vi "总磷总氮流程质控自动启动.vi"(9 "总磷量程切换":enum32{"H", "L", "AUTO"}(ring)=enum."AUTO", 10 "总氮量程切换":enum32{"H", "L", "AUTO"}(ring)=enum."AUTO", 11 "参数":T1={"是否启用仪器"=FALSE, "CODMn"={"启动测量模式"={"测量模式"=enum."水样测量"}, "确定按钮"=TRUE}, "启动模块"={"氨氮"=FALSE, "总磷"=FALSE, "总氮"=FALSE, "COD"=FALSE}, "常规启动"=FALSE, "直接启动"=FALSE}) -> ()   [LabVIEW 2016, in "质控单元.lvlib"]
uses:
  PLC/PLC.lvlib
panel:
  out "枚举 2":enum16{"初始化", "采配水启动", "等待", "配水", "排水", "结束"}(ring)
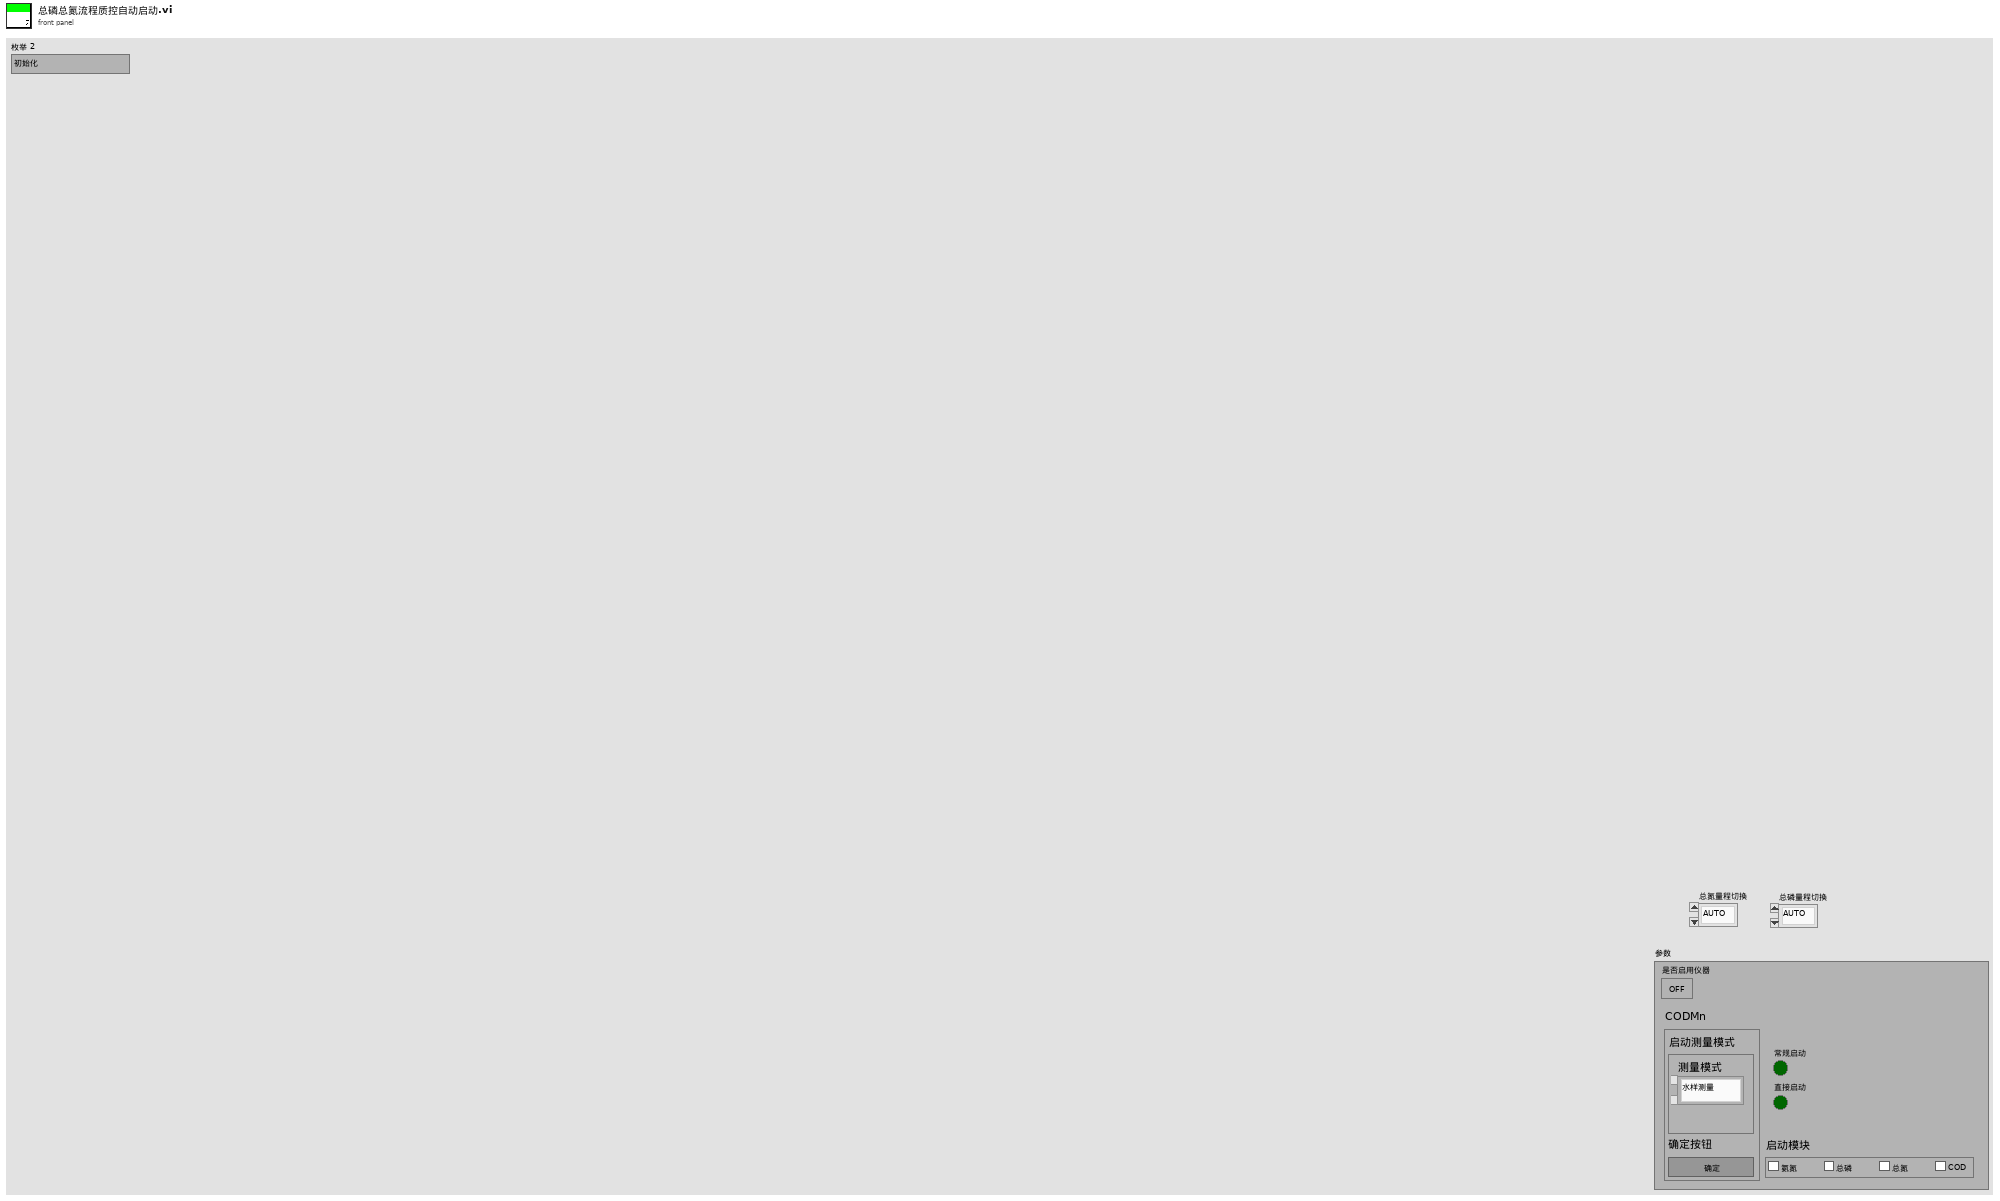
[diagram p1: front panel]
types:
  T1 = cluster{"是否启用仪器":bool, "CODMn":cluster{"启动测量模式":cluster{"测量模式":enum16{"水样测量", "标样核查", "加标回收", "平行样", "校零", "校标"}}, "确定按钮":bool}, "启动模块":cluster{"氨氮":bool, "总磷":bool, "总氮":bool, "COD":bool}, "常规启动":bool, "直接启动":bool}
  T2 = cluster{"R0":i16, "R1":i16, "R2":i16, "R3":i16, "R4":i16, "R5":i16, "R6":i16, "R7":i16, "R8":i16, "R9":i16, "R10":i16, "R11":i16, "R12":i16, "R13":i16, "R14":i16, "R15":i16, "R16":i16, "R17":i16, "R18":i16, "R19":i16, "R20":i16, "R21":i16, "R22":i16, "R23":i16, "R24":i16, "R25":i16, "R26":i16, "R27":i16, "R28":i16, "R29":i16, "R30":i16, "R31":i16, "R32":i16, "R33":i16, "R34":i16, "R35":i16, "R36":i16, "R37":i16, "R38":i16, "R39":i16, "R40":i16, "R41":i16, "R42":i16, "R43":i16, "R44":i16, "R45":i16, "R46":i16, "R47":i16, "R48":i16, "R49":i16, "R50":i16, "R51":i16, "R52":i16, "R53":i16, "R54":i16, "R55":i16, "R56":i16}
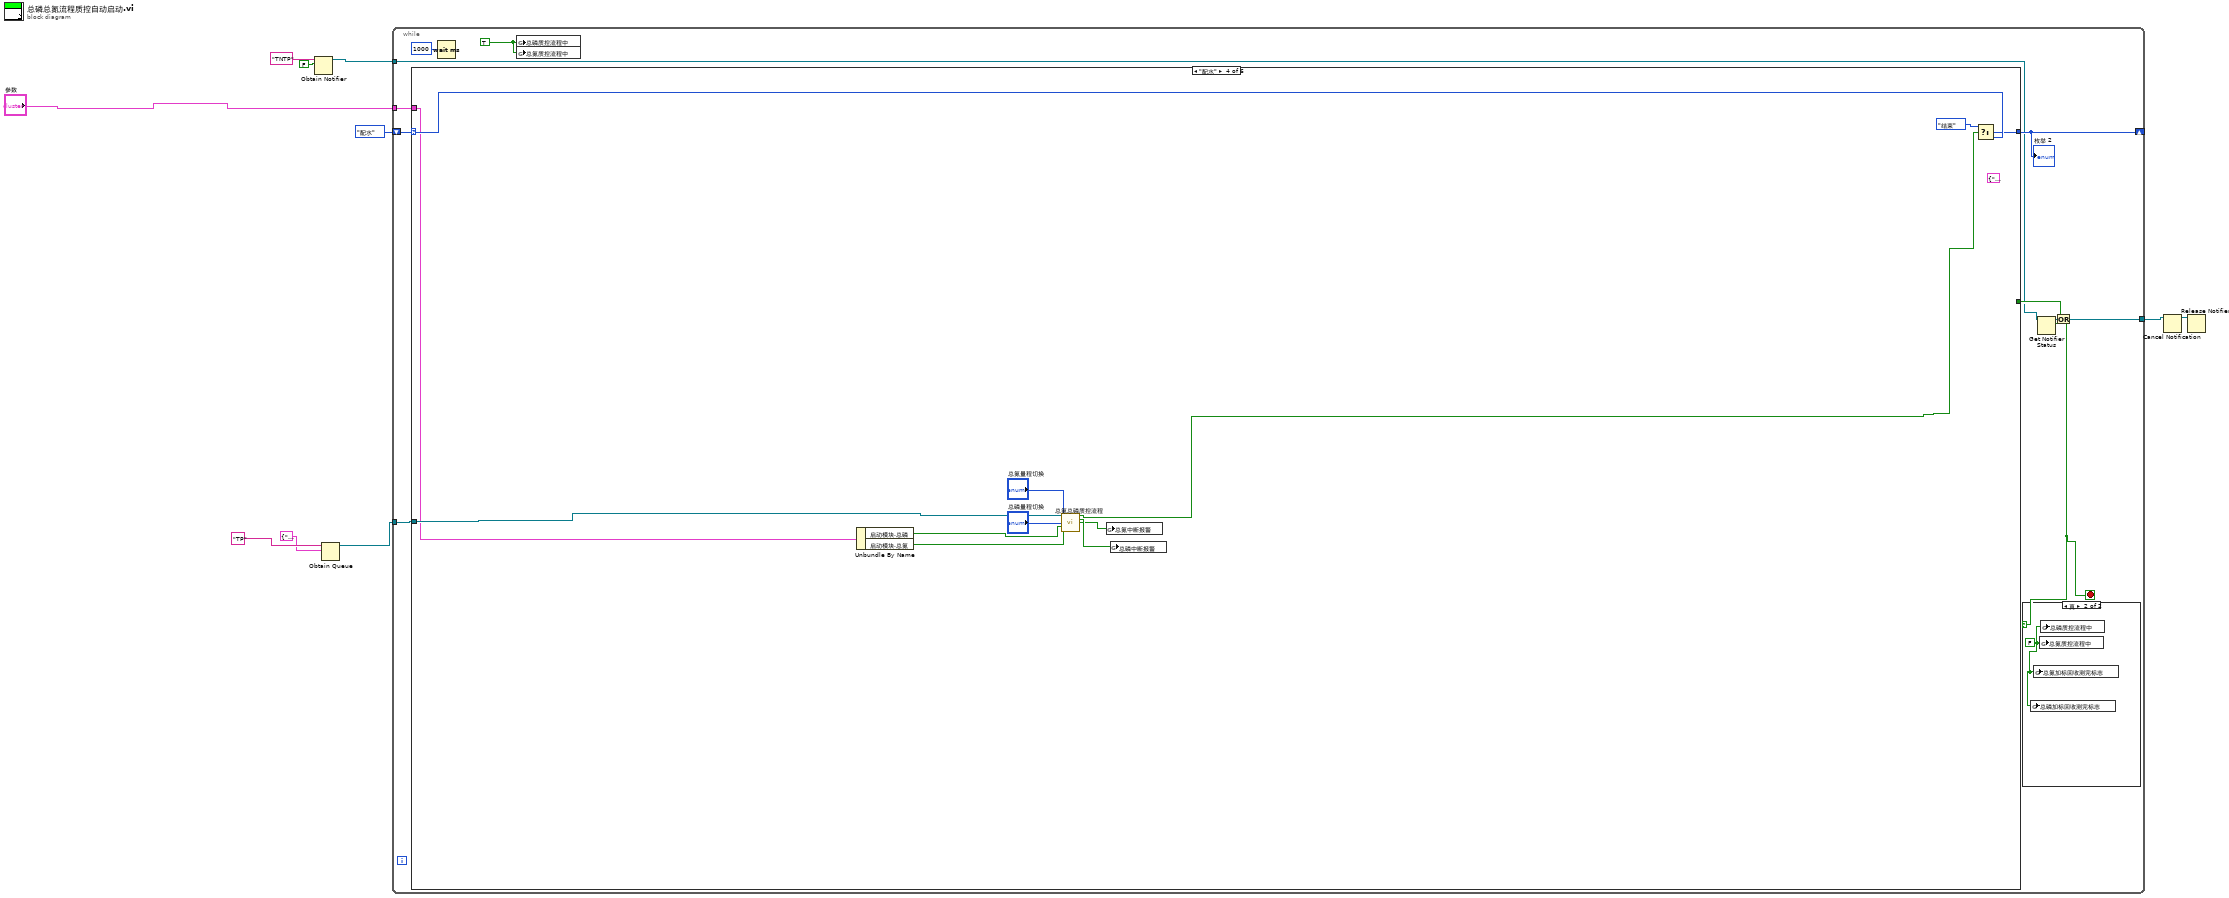
[diagram p0: block diagram]
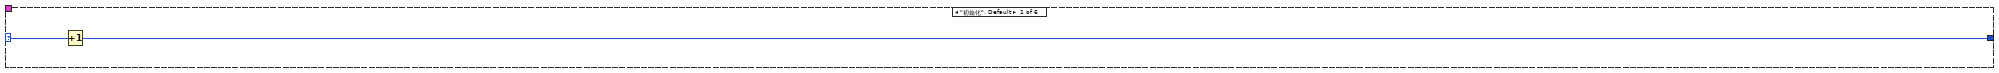
[diagram p3: hidden frame]
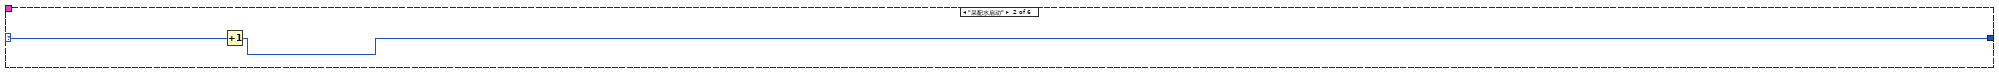
[diagram p4: hidden frame]
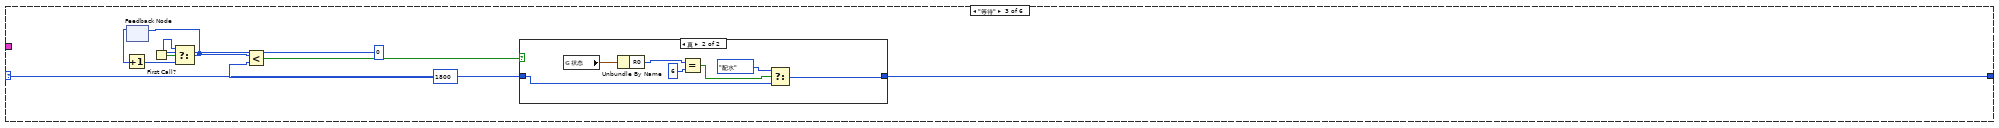
[diagram p5: hidden frame]
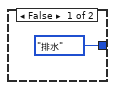
[diagram p6: hidden frame]
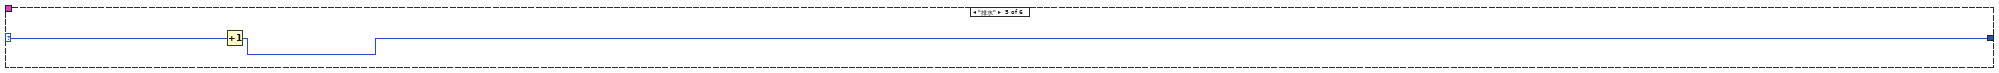
[diagram p7: hidden frame]
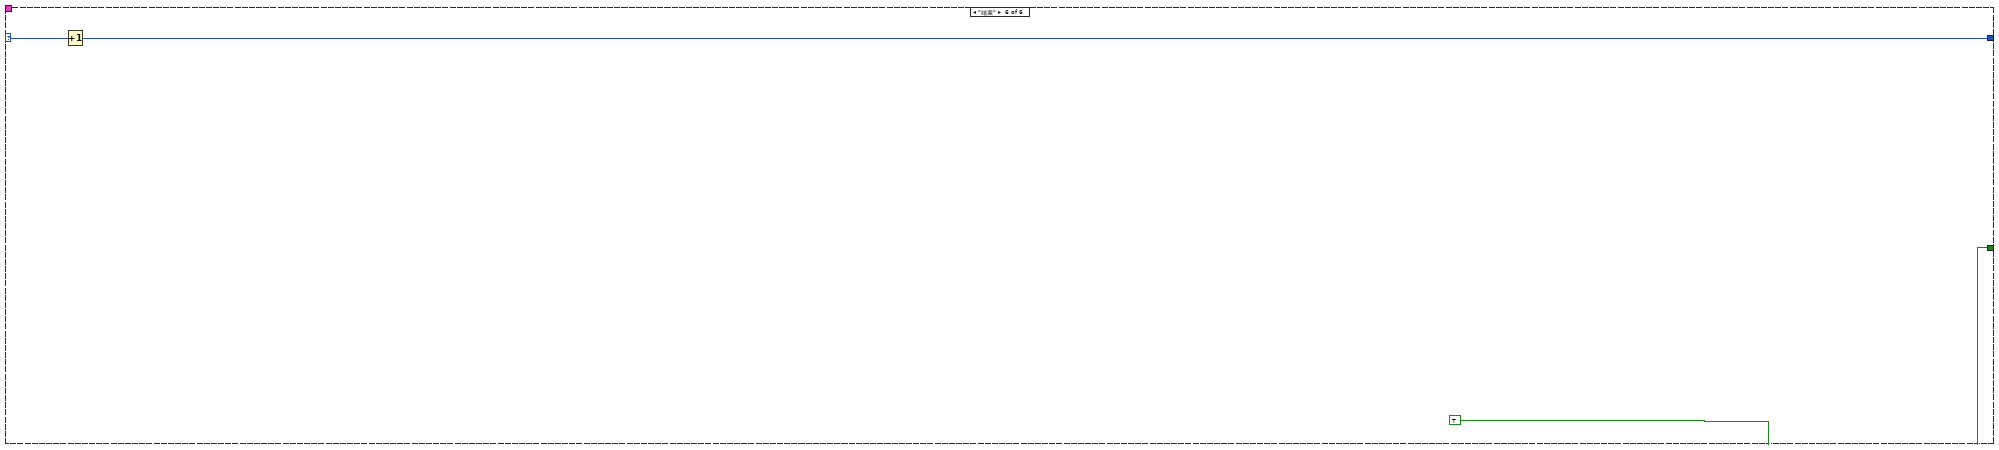
[diagram p8: hidden frame]
diagram:
  n1 = Obtain Notifier(name (unnamed)="TNTP" ("名称（未命名）"), notification data type=FALSE) -> (notifier out=w3:refnum<notifier>)  [unwired: 2 in, 2 out]
  n2 = Obtain Queue(name (unnamed)="TP" ("名称（未命名）"), element data type=cluster{"命令":string, "data":variant} {"命令"="", "data"=variant}) -> (queue out=w6:refnum<queue>)  [unwired: 3 in, 2 out]
  n3 = while {
    shift-right: [w20] -> _
    shift-left: enum16{"初始化", "采配水启动", "等待", "配水", "排水", "结束"}."配水" ("枚举") -> [w21]
    tunnel: w6 -> [w18]
    tunnel: "参数" -> [w17]
    tunnel: w3 -> [w14]
    tunnel: [w13] -> w1
    stop <- w11 stop-if-true
    w12 = TRUE ("总磷质控流程中")
    n4 = case shown="\"配水\"" w21 {
      selector: w21 -> [w24 w26 w33 w54 w57 w60]
      tunnel: [w23 w25 w32 w53 w56 w59] -> w20
      tunnel: [_ _ _ _ _ TRUE] -> w16
      tunnel: w18 -> [_ _ _ w52 _ _]
      tunnel: w17 -> [_ _ _ w46 _ _]
      frame "初始化", Default {
        n5 = Increment(x=w24) -> (x+1=w23:enum16{"初始化", "采配水启动", "等待", "配水", "排水", "结束"})
      }
      frame "采配水启动" {
        n6 = Increment(x=w26) -> (x+1=w25:enum16{"初始化", "采配水启动", "等待", "配水", "排水", "结束"})
      }
      frame "等待" {
        n7 = feedback #1() -> (w29:i32)  [unwired: 1 in]
        n8 = Increment(x=w29) -> (x+1=w28:i32)
        n9 = First Call?() -> (First Call?: T/F=w30:bool)
        n10 = Select(t=0, s=w30, f=w28) -> (s? t:f=w27:i32)
        n11 = feedback-in #1(w27) -> ()
        n12 = Less?(x=w27, y=1800) -> (x < y?=w34:bool)
        n13 = case shown="真" w34 {
          tunnel: w33 -> [_ w38]
          tunnel: [enum16{"初始化", "采配水启动", "等待", "配水", "排水", "结束"}."排水" ("枚举") w37] -> w32
          frame False {
          }
          frame True {
            n14 = global read "采配水全局变量.vi" "状态"() -> (w43:T2)
            n15 = Unbundle By Name(w43) -> ("R0"=w42:i16)
            n16 = Equal?(x=w42, y=i16 6) -> (x = y?=w40:bool)
            n17 = Select(t=enum16{"初始化", "采配水启动", "等待", "配水", "排水", "结束"}."配水" ("枚举"), s=w40, f=w38) -> (s? t:f=w37:enum16{"初始化", "采配水启动", "等待", "配水", "排水", "结束"})
          }
        }
      }
      frame "配水" {
        (unwired) cluster{"命令":string, "data":variant} {"命令"="启动", "data"=variant(cluster{"站号":u16, "控制命令输出":u16[]} {"站号"=1, "控制命令输出"=[256, 0]})} ("元素")
        n18 = Unbundle By Name(w46) -> ("启动模块.总磷"=w45:bool, "启动模块.总氮"=w44:bool)
        n19 = call "总氮总磷质控流程.vi"("队列输入TP"=w52, "总氮量程切换"="总氮量程切换", "总磷量程切换"="总磷量程切换", "总磷"=w45, "总氮"=w44) -> ("布尔"=w49:bool, "总磷中断报警"=w48:bool, "总氮中断报警"=w47:bool)  [unwired: 8 in]
        n20 = global write "质控中断报警全局.vi" "总氮中断报警"(w47) -> ()
        n21 = global write "质控中断报警全局.vi" "总磷中断报警"(w48) -> ()
        n22 = Select(t=enum16{"初始化", "采配水启动", "等待", "配水", "排水", "结束"}."结束" ("枚举"), s=w49, f=w54) -> (s? t:f=w53:enum16{"初始化", "采配水启动", "等待", "配水", "排水", "结束"})
      }
      frame "排水" {
        n23 = Increment(x=w57) -> (x+1=w56:enum16{"初始化", "采配水启动", "等待", "配水", "排水", "结束"})
      }
      frame "结束" {
        n24 = Increment(x=w60) -> (x+1=w59:enum16{"初始化", "采配水启动", "等待", "配水", "排水", "结束"})
      }
    }
    "枚举 2" <- w20
    n25 = Wait (ms)(milliseconds to wait=u32 1000 ("等待时间（毫秒）")) -> ()  [unwired: 1 out]
    n26 = global write "质控测完标志全局 1.vi" "总磷质控流程中"(w12) -> ()
    n27 = global write "质控测完标志全局 1.vi" "总氮质控流程中"(w12) -> ()
    n28 = Get Notifier Status(notifier=w14) -> (notifier out=w13:refnum<notifier>, current notification=w15:bool)  [unwired: 1 in, 3 out]
    n29 = Or(x=w16, y=w15) -> (x .or. y?=w11:bool)
    n30 = case shown="真" w11 {
      frame False {
      }
      frame True {
        w22 = FALSE ("总氮质控流程中")
        n31 = global write "质控测完标志全局 1.vi" "总磷加标回收测完标志"(w22) -> ()
        n32 = global write "质控测完标志全局 1.vi" "总氮加标回收测完标志"(w22) -> ()
        n33 = global write "质控测完标志全局 1.vi" "总氮质控流程中"(w22) -> ()
        n34 = global write "质控测完标志全局 1.vi" "总磷质控流程中"(w22) -> ()
      }
    }
  }
  n35 = Cancel Notification(0:w1) -> (8:w2:refnum<notifier>)  [unwired: 1 in, 2 out]
  n36 = Release Notifier(notifier=w2) -> ()  [unwired: 2 in, 3 out]
